vi "get all files.vi"() -> ()   [LabVIEW 2009]
panel:
  out "Array":path[](array[path])
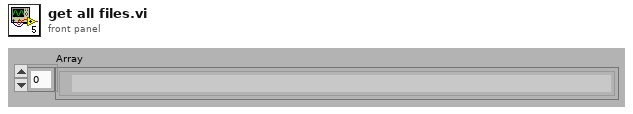
[diagram p1: front panel]
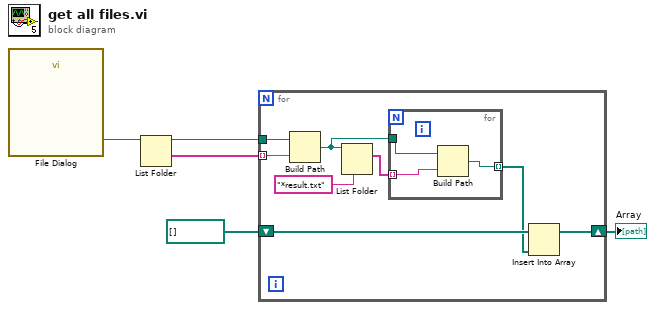
[diagram p0: block diagram]
diagram:
  n1 = call "File Dialog"() -> ("selected path"=w5:path)  [unwired: 12 in, 3 out]
  n2 = List Folder(path=w5) -> (path out=w3:path, folder names=w4:string[])  [unwired: 3 in, 2 out]
  n3 = for {
    tunnel: w4 -> [w12] mode=indexing
    tunnel: w3 -> [w13]
    shift-right: [w6] -> w1
    shift-left: path[] [] -> [w8]
    n4 = Build Path(base path=w13, name or relative path=w12) -> (appended path=w11:path)
    n5 = List Folder(path=w11, pattern="*result.txt") -> (filenames=w10:string[])  [unwired: 2 in, 3 out]
    n6 = for {
      tunnel: w11 -> [w16]
      tunnel: w10 -> [w15] mode=indexing
      tunnel: [w14] -> w7 mode=indexing
      n7 = Build Path(base path=w16, name or relative path=w15) -> (appended path=w14:path)
    }
    n8 = Insert Into Array(array=w8, new element=w7) -> (w6:path[])  [unwired: 1 in]
  }
  "Array" <- w1
